vi "signal_spectrum.vi"() -> ()   [LabVIEW 2024]
uses:
  <vilib>/sound2/lvsound2.llb/Sound Data Format.ctl
  <vilib>/sound2/lvsound2.llb/Sampling Mode.ctl
  <vilib>/sound2/lvsound2.llb/Sound Input Read (DBL).vi
  <vilib>/measure/maspectr.llb/FFT Spectrum (Mag-Phase) for N Chan.vi
  <vilib>/measure/NI_MAPro.lvlib
panel:
  out "Stroik":T1
  out "Note":dbl
  out "Highest freq":dbl
  out "error out":errorcluster
  out "Intensity Chart":dbl[][](graph)
  out "Waveform Graph":cluster{"f0":dbl, "df":dbl, "magnitude":dbl[]}[](graph)
  in  "device ID":u32
  in  "stop":bool
  in  "sound format":T2={"sample rate (S/s)"=22050.0, "number of channels"=2, "bits per sample"=16}
  out "test2":waveform(dbl)[](graph)
  out "test":cluster{"f0":dbl, "df":dbl, "magnitude":dbl[]}[](graph)
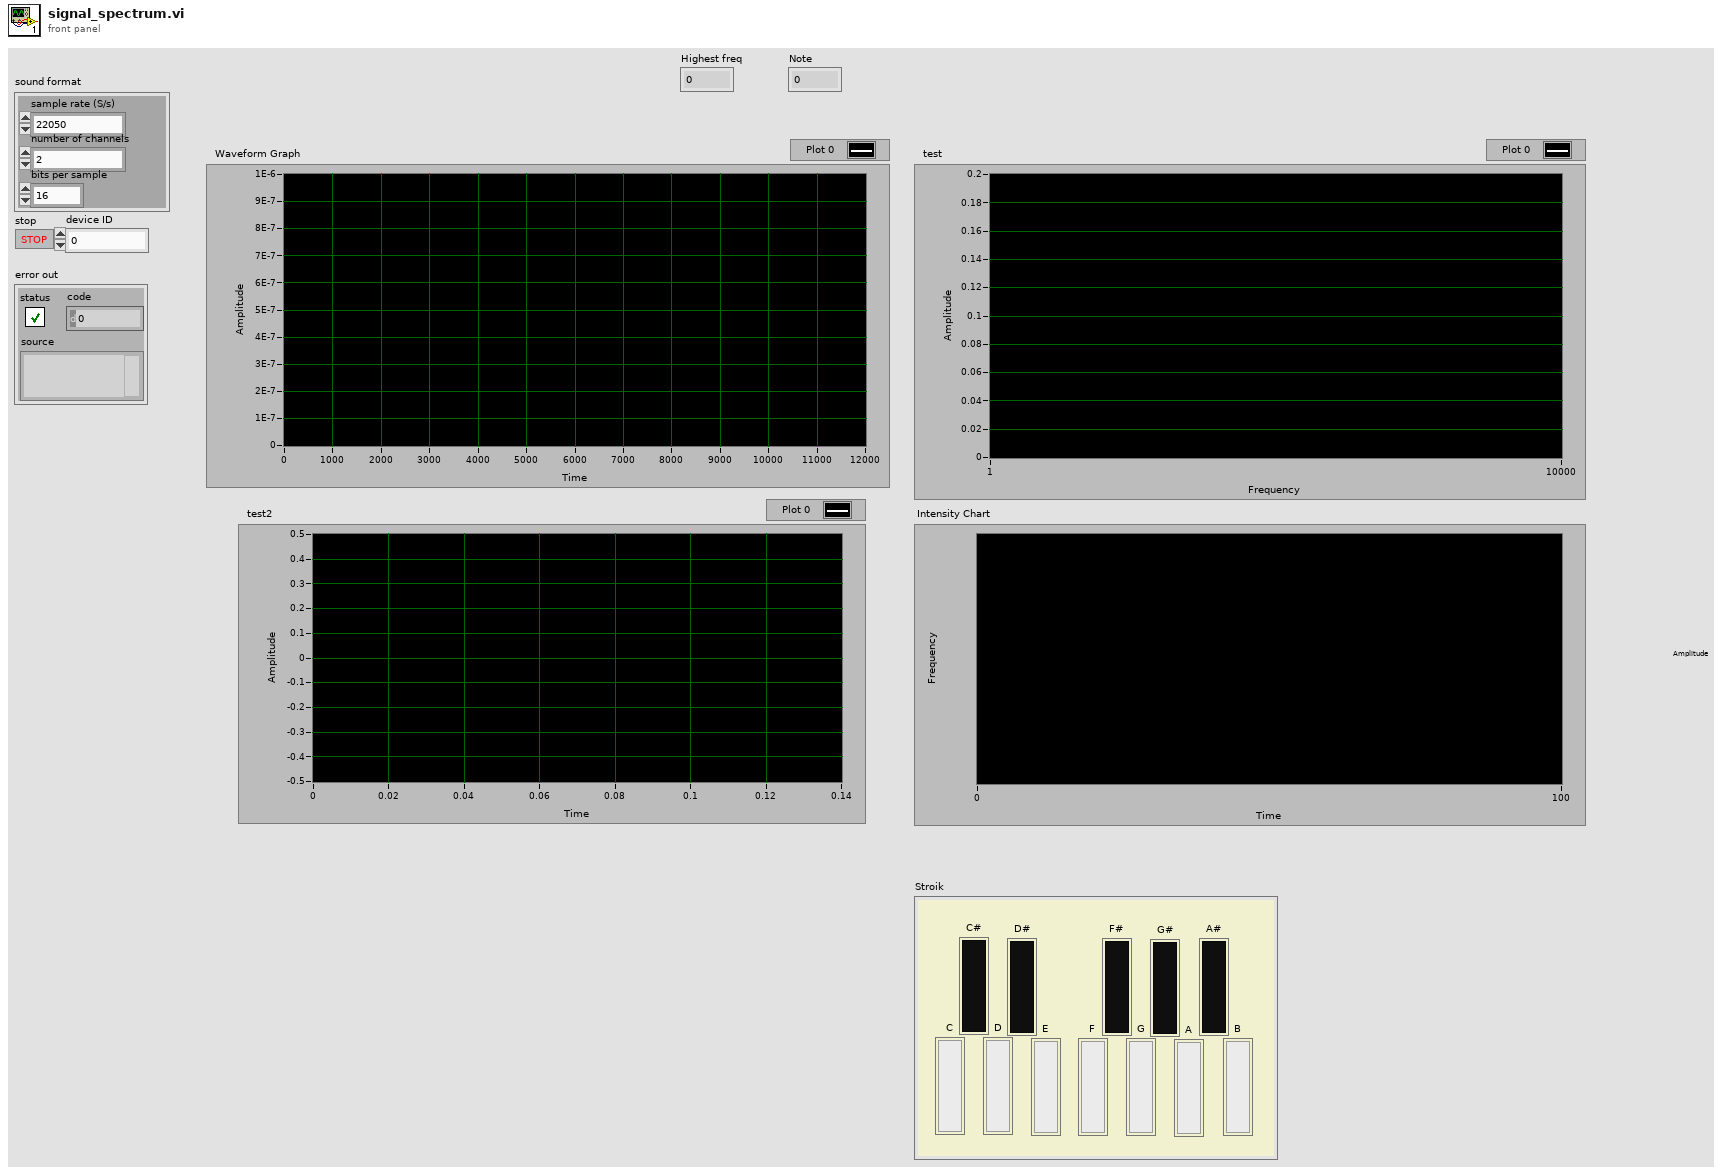
[diagram p1: front panel]
types:
  T1 = cluster{"A":bool, "A#":bool, "B":bool, "C":bool, "C#":bool, "D":bool, "D#":bool, "E":bool, "F":bool, "F#":bool, "G":bool, "G#":bool}
  T2 = typedef "Sound Data Format.ctl" = cluster{"sample rate (S/s)":dbl, "number of channels":i32, "bits per sample":i32}
  T3 = typedef "Sampling Mode.ctl" = i32
  T4 = typedef "Sound Input Task ID.ctl" = u32
  T5 = cluster{"[0]":bool, "[1]":bool, "[2]":bool, "[3]":bool, "[4]":bool, "[5]":bool, "[6]":bool, "[7]":bool, "[8]":bool, "[9]":bool, "[10]":bool, "[11]":bool}
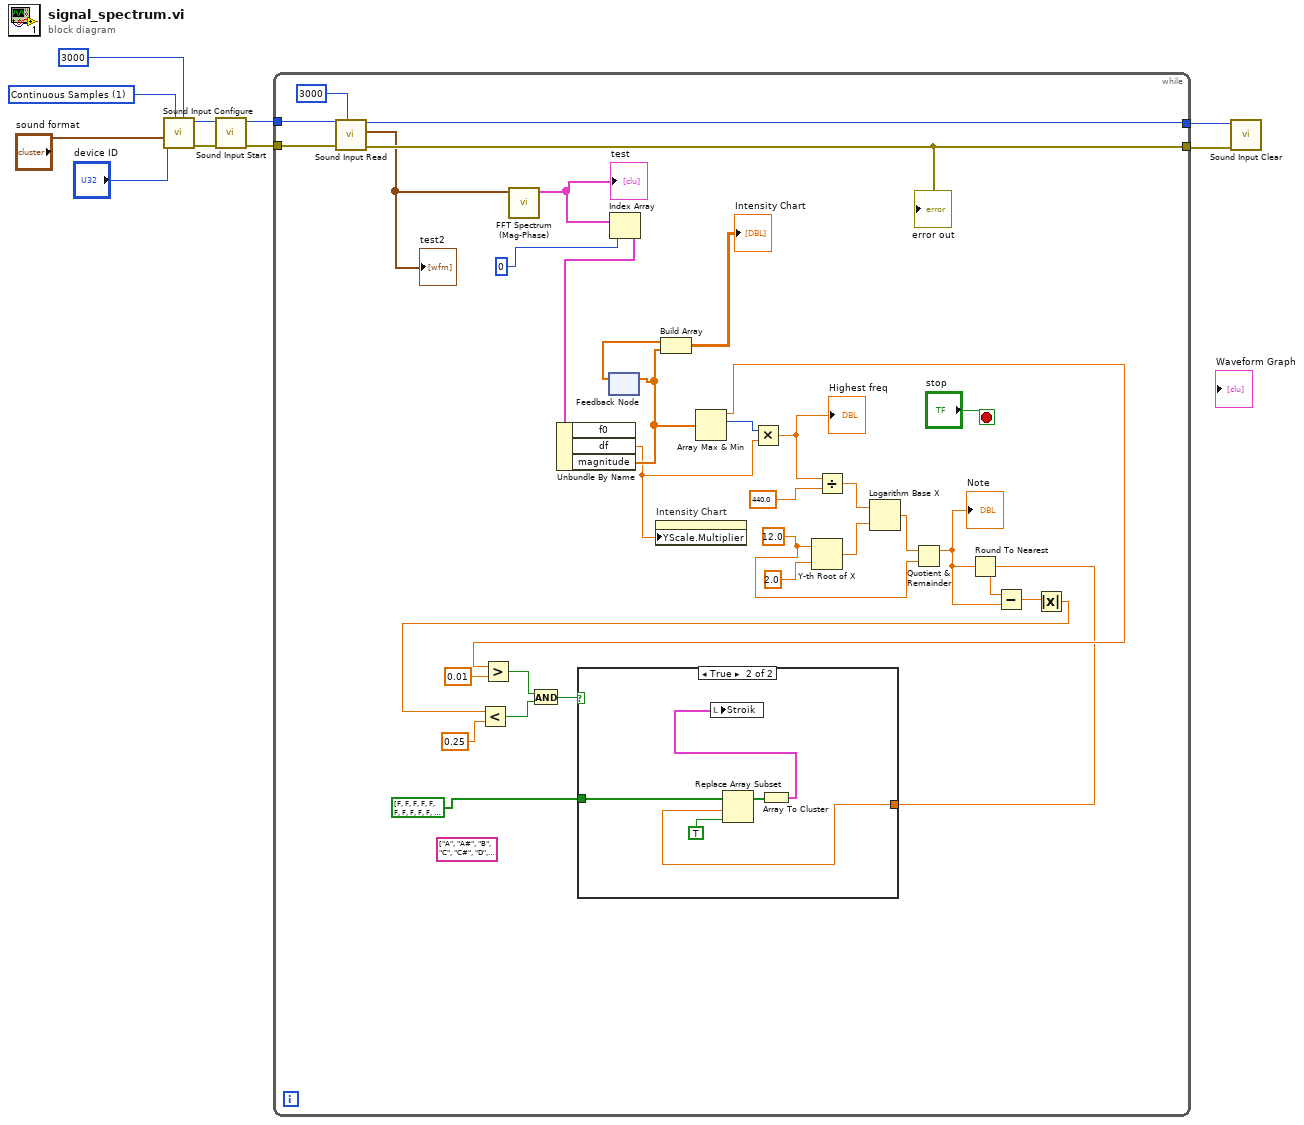
[diagram p0: block diagram]
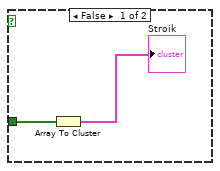
[diagram p2: hidden frame]
diagram:
  w10 = T3 1 items=["Finite Samples", "Continuous Samples"] ("sample mode")
  n1 = call <vilib>:"Sound Input Configure.vi"("number of samples/ch"=3000, "sample mode"=w10, "sound format"="sound format", "device ID"="device ID") -> ("error out"=w2:errorcluster, "task ID"=w8:T4)  [unwired: 6 in]
  n2 = call <vilib>:"Sound Input Start.vi"("error in (no error)"=w2, "task ID"=w8) -> ("error out"=w1:errorcluster, "task ID out"=w7:T4)  [unwired: 8 in]
  n3 = while {
    tunnel: w7 -> [w42]
    tunnel: w1 -> [w41]
    tunnel: [w39] -> w6
    tunnel: [w38] -> w5
    stop <- "stop" stop-if-true
    (unwired) string[] ["A", "A#", "B", "C", "C#", "D", "D#", "E", "F", "F#", "G", "G#"]
    w22 = 12.0 ("y")
    n4 = call-poly <vilib>:"Sound Input Read.vi"("number of samples/ch"=3000, "error in (no error)"=w41, "task ID"=w42) -> ("error out"=w38:errorcluster, "data"=w37:waveform(dbl)[], "task ID out"=w39:T4)  [unwired: 6 in]
    "test2" <- w37
    "error out" <- w38
    n5 = call-poly <vilib>:"FFT Spectrum (Mag-Phase).vi"("time signals"=w37) -> ("magnitudes"=w34:cluster{"f0":dbl, "df":dbl, "magnitude":dbl[]}[])  [unwired: 6 in, 4 out]
    "test" <- w34
    n6 = feedback #1() -> (w32:dbl[])  [unwired: 1 in]
    n7 = Index Array(array=w34, index=0) -> (element=w35:cluster{"f0":dbl, "df":dbl, "magnitude":dbl[]})
    n8 = Unbundle By Name(w35) -> ("df"=w29:dbl, "magnitude"=w31:dbl[])  [unwired: 1 out]
    n9 = feedback-in #1(w31) -> ()
    n10 = property on="Intensity Chart" class="IntChart (strict)"("YScale.Multiplier"=w29) -> ()  [unwired: 2 in, 2 out]
    n11 = Build Array(w32, w31) -> (→"Intensity Chart":dbl[][])
    n12 = Array Max & Min(array=w31) -> (max value=w18:dbl, max index (indices)=w30:i32)  [unwired: 2 out]
    n13 = Greater?(x=w18, y=0.01) -> (0:w16:bool)
    n14 = Multiply(x=w30, y=w29) -> (x*y=w28:dbl)
    "Highest freq" <- w28
    n15 = Y-th Root of X(1:2.0 ("x"), 2:w22) -> (0:w24:dbl)
    n16 = Divide(x=w28, y=440.0) -> (x/y=w26:dbl)
    n17 = Logarithm Base X(1:w24, 2:w26) -> (0:w23:dbl)
    n18 = Quotient & Remainder(x=w23, y=w22) -> (x-y*floor(x/y)=w21:dbl)  [unwired: 1 out]
    "Note" <- w21
    n19 = Round To Nearest(number=w21) -> (nearest integer value=w12:dbl)
    n20 = Subtract(x=w12, y=w21) -> (x-y=w20:dbl)
    n21 = Absolute Value(x=w20) -> (abs(x)=w15:dbl)
    n22 = Less?(x=w15, y=0.25) -> (x < y?=w13:bool)
    n23 = And(x=w16, y=w13) -> (x .and. y?=w19:bool)
    n24 = case shown="True" w19 {
      tunnel: w12 -> [_ w48]
      tunnel: bool[] [FALSE, FALSE, FALSE, FALSE, FALSE, FALSE, FALSE, FALSE, FALSE, FALSE, FALSE, FALSE, FALSE] -> [w44 w50]
      frame False {
        n25 = Array To Cluster(array=w44) -> (cluster=→"Stroik":T5)
      }
      frame True {
        n26 = Replace Array Subset(array=w50, new element=TRUE, index=w48) -> (w47:bool[])
        n27 = Array To Cluster(array=w47) -> (cluster=w46:T5)
        n28 = local write "Stroik"(w46) -> ()
      }
    }
  }
  n29 = call <vilib>:"Sound Input Clear.vi"("error in (no error)"=w5, "task ID"=w6) -> ()  [unwired: 9 in, 1 out]
